vi "ReadValue_DBL.vi"(11 "reference":refnum<vi>) -> (2 "value":dbl)   [LabVIEW 2012]
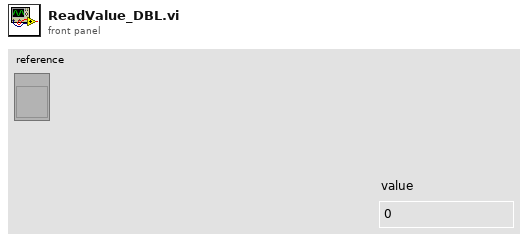
[diagram p1: front panel]
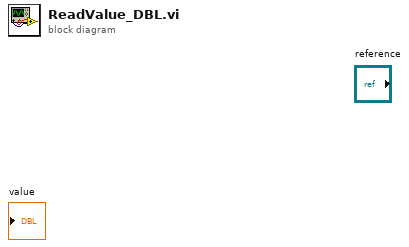
[diagram p0: block diagram]
diagram:
